vi "Display Tree Item.vi"(8 "error in (no error)":errorcluster, 10 "Tag":string, 11 "Application Data in":T1) -> (0 "error out":errorcluster, 3 "Application Data out":T1)   [LabVIEW 2017, in "DSF Configuration Utility.lvlib"]
uses:
  DSF Configuration Utility.lvlib
  Application Data.ctl
  VeriStand/Data Sharing Custom Device/Source/Engine/DSF Core.lvlibp/Classes/Configuration/Configuration Session.lvclass
  View Mode.ctl
  VeriStand/Data Sharing Custom Device/Source/Engine/DSF Core.lvlibp/Classes/Configuration/Read Plugin.vi
  VeriStand/Data Sharing Custom Device/Source/Engine/DSF Core.lvlibp/Classes/Configuration/Read Settings.vi
  VeriStand/Data Sharing Custom Device/Source/Engine/DSF Core.lvlibp/Classes/Configuration/Read Channel.vi
  VeriStand/Data Sharing Custom Device/Source/Engine/DSF Core.lvlibp/Classes/Configuration/Read Transfer.vi
  VeriStand/Data Sharing Custom Device/Source/Engine/DSF Core.lvlibp/Classes/Configuration/Read Group.vi
panel:
  # "App\nData"
  # "App\nData"
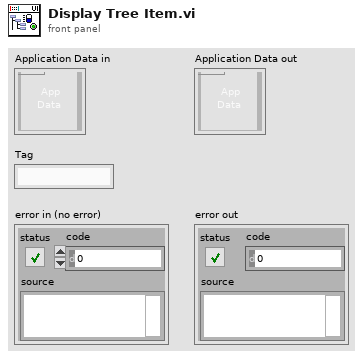
[diagram p1: front panel]
types:
  T1 = typedef "DSF Configuration Utility.lvlib/Application Data.ctl" = cluster{"Item Tree Control":refnum<vi>, "Value Tree Control":refnum<vi>, "DSF Refnum":refnum<class "Configuration Session.lvclass">, "Top-Level VI":refnum<vi>, "View State":T2, "menu reference":refnum<k9>}
  T2 = typedef "DSF Configuration Utility.lvlib/View Mode.ctl" = enum16{"Tree", "List"}
  T3 = typedef "DSF Core.lvlibp/DSF Version Info.ctl" = cluster{"major":u32, "minor":u32, "fix":u32, "build":string}
  T4 = typedef "DSF Configuration Utility.lvlib/Tree Item Type.ctl" = enum16{"Plugin", "Group", "Transfer", "Channel", "Setting"}
  T5 = typedef "DSF Core.lvlibp/DSF Group Info.ctl" = cluster{"direction":T6, "timing":T7, "transfer ids":string[], "settings id":string, "thread":i32}
  T6 = typedef "DSF Core.lvlibp/DSF Direction.ctl" = enum8{"Tx", "Rx"}
  T7 = typedef "DSF Core.lvlibp/DSF Timing Info.ctl" = cluster{"priority":u64, "decimation":u64, "offset":u64}
  T8 = typedef "DSF Core.lvlibp/DSF Transfer Info.ctl" = cluster{"byte order":T9, "channel ids":string[], "settings id":string}
  T9 = typedef "DSF Core.lvlibp/DSF Byte Order.ctl" = enum8{"big-endian", "little-endian"}
  T10 = typedef "DSF Core.lvlibp/DSF Channel Info.ctl" = cluster{"string buffer offset":u64, "string data type":T11, "engine data type":T11, "settings id":string}
  T11 = typedef "DSF Core.lvlibp/DSF Data Type.ctl" = enum8{"Bool", "SGL", "DBL", "I8", "I16", "I32", "I64", "U8", "U16", "U32", "U64"}
  T12 = typedef "DSF Core.lvlibp/DSF Settings Info.ctl" = cluster{"key":string, "value":string}[]
  T13 = typedef "DSF Core.lvlibp/DSF Plugin Info.ctl" = cluster{"components":string[], "timing":T7, "group ids":string[], "settings id":string, "threads":T14[]}
  T14 = typedef "DSF Core.lvlibp/DSF Engine Plugin Thread Configuration.ctl" = cluster{"buffer converter settings":T12, "transceiver settings":T12, "processor":i32}
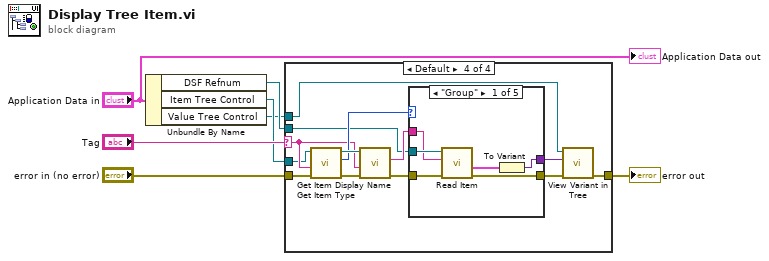
[diagram p0: block diagram]
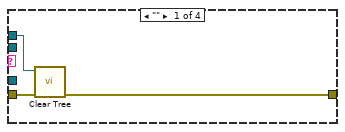
[diagram p2: hidden frame]
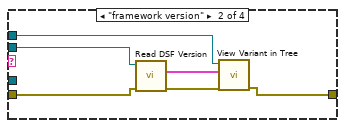
[diagram p3: hidden frame]
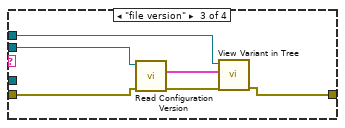
[diagram p4: hidden frame]
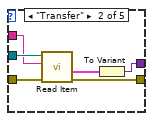
[diagram p5: hidden frame]
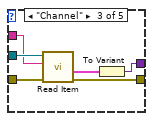
[diagram p6: hidden frame]
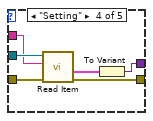
[diagram p7: hidden frame]
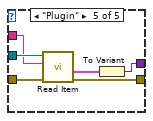
[diagram p8: hidden frame]
diagram:
  n1 = Unbundle By Name("Application Data in") -> ("DSF Refnum"=w5:refnum<class "Configuration Session.lvclass">, "Item Tree Control"=w4:refnum<vi>, "Value Tree Control"=w2:refnum<vi>)
  n2 = case shown="Default" "Tag" {
    selector: "Tag" -> [_ _ _ w30]
    tunnel: w5 -> [_ w16 w22 w29]
    tunnel: w4 -> [_ _ _ w28]
    tunnel: "error in (no error)" -> [w10 w15 w21 w27]
    tunnel: w2 -> [w8 w11 w17 w24]
    tunnel: [w9 w13 w19 w23] -> w1
    frame "" {
      n3 = call "Clear Tree.vi"("error in (no error)"=w10, "TreeControl in"=w8) -> ("error out"=w9:errorcluster)  [unwired: 9 in]
    }
    frame "framework version" {
      n4 = call "Read DSF Version.vi"("error in (no error)"=w15, "Configuration Session in"=w16) -> ("error out"=w14:errorcluster, "dsfversion"=w12:T3)  [unwired: 7 in, 1 out]
      n5 = call "View Variant in Tree.vi"("error in (no error)"=w14, "Variant"=w12, "TreeControl in"=w11) -> ("error out"=w13:errorcluster)  [unwired: 8 in]
    }
    frame "file version" {
      n6 = call "Read Configuration Version.vi"("error in (no error)"=w21, "Configuration Session in"=w22) -> ("error out"=w20:errorcluster, "version"=w18:T3)  [unwired: 7 in, 1 out]
      n7 = call "View Variant in Tree.vi"("error in (no error)"=w20, "Variant"=w18, "TreeControl in"=w17) -> ("error out"=w19:errorcluster)  [unwired: 8 in]
    }
    frame Default {
      n8 = call "Get Item Type.vi"("error in (no error)"=w27, "Tag"=w30, "TreeControl in"=w28) -> ("error out"=w34:errorcluster, "Item Type"=w32:T4, "TreeControl out"=w33:refnum<vi>)  [unwired: 6 in]
      n9 = call "Get Item Display Name.vi"("error in (no error)"=w34, "Tag"=w30, "TreeControl in"=w33) -> ("error out"=w35:errorcluster, "display name"=w31:string)  [unwired: 6 in, 1 out]
      n10 = case shown="\"Group\"" w32 {
        tunnel: w31 -> [w36 w42 w48 w54 w60]
        tunnel: [w40 w45 w51 w58 w64] -> w26
        tunnel: w35 -> [w39 w46 w52 w59 w65]
        tunnel: w29 -> [w38 w44 w50 w57 w63]
        tunnel: [w37 w43 w49 w55 w62] -> w25
        frame "Group" {
          n11 = call-poly "Read Item.vi"("error in (no error)"=w39, "Group ID"=w36, "Configuration Session in"=w38) -> ("error out"=w40:errorcluster, "value"=w41:T5)  [unwired: 5 in, 2 out]
          n12 = To Variant(anything=w41) -> (Variant=w37:variant)
        }
        frame "Transfer" {
          n13 = call-poly "Read Item.vi"("error in (no error)"=w46, "Transfer ID"=w42, "Configuration Session in"=w44) -> ("error out"=w45:errorcluster, "value"=w47:T8)  [unwired: 5 in, 2 out]
          n14 = To Variant(anything=w47) -> (Variant=w43:variant)
        }
        frame "Channel" {
          n15 = call-poly "Read Item.vi"("error in (no error)"=w52, "Channel ID"=w48, "Configuration Session in"=w50) -> ("error out"=w51:errorcluster, "value"=w53:T10)  [unwired: 5 in, 2 out]
          n16 = To Variant(anything=w53) -> (Variant=w49:variant)
        }
        frame "Setting" {
          n17 = call-poly "Read Item.vi"("error in (no error)"=w59, "Settings ID"=w54, "Configuration Session in"=w57) -> ("error out"=w58:errorcluster, "value"=w56:T12)  [unwired: 5 in, 2 out]
          n18 = To Variant(anything=w56) -> (Variant=w55:variant)
        }
        frame "Plugin" {
          n19 = call-poly "Read Item.vi"("error in (no error)"=w65, "Plugin ID"=w60, "Configuration Session in"=w63) -> ("error out"=w64:errorcluster, "value"=w61:T13)  [unwired: 5 in, 2 out]
          n20 = To Variant(anything=w61) -> (Variant=w62:variant)
        }
      }
      n21 = call "View Variant in Tree.vi"("error in (no error)"=w26, "Variant"=w25, "TreeControl in"=w24) -> ("error out"=w23:errorcluster)  [unwired: 8 in]
    }
  }
  "error out" <- w1
  "Application Data out" <- "Application Data in"
